vi "Initialize.vi"(7 "Parcel Weight [kg]":dbl, 8 "error in (no error)":errorcluster, 9 "Recipient Data":T1, 10 "Sender Data":T1, 11 "Courier in":refnum<class "Courier.lvclass">) -> (0 "error out":errorcluster, 3 "Courier out":refnum<class "Courier.lvclass">)   [LabVIEW 2019, in "Courier.lvclass"]
uses:
  Courier.lvclass
  C:/Users/Extensa/Desktop/Fabryka/Fabryka Rozwiazanie/Delivery/Delivery/Delivery.lvclass
  Controls/#cluster_PersonalData.ctl
  Delivery/Delivery.lvclass/Delivery.ctl
  Delivery/Delivery.lvclass
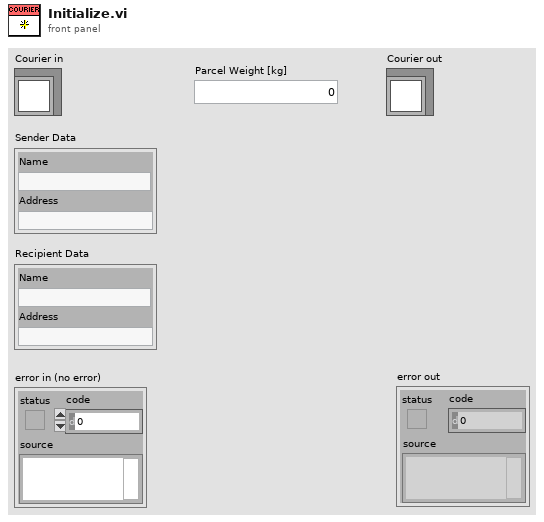
[diagram p1: front panel]
types:
  T1 = typedef "#cluster_PersonalData.ctl" = cluster{"Name":string, "Address":string}
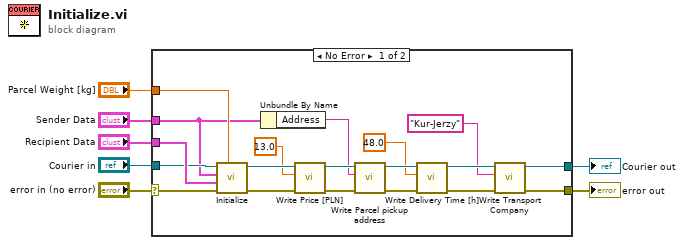
[diagram p0: block diagram]
diagram:
  n1 = case shown="No Error" "error in (no error)" {
    selector: "error in (no error)" -> [w25 w27]
    tunnel: [w8 w27] -> w7
    tunnel: [w9 w28] -> w6
    tunnel: "Parcel Weight [kg]" -> [w26 _]
    tunnel: "Recipient Data" -> [w24 _]
    tunnel: "Sender Data" -> [w17 _]
    tunnel: "Courier in" -> [w23 w28]
    frame No Error {
      n2 = call-parent "Initialize.vi"("Parcel Weight [kg]"=w26, "error in (no error)"=w25, "Recipient Data"=w24, "Sender Data"=w17, "Delivery in"=w23) -> ("error out"=w21:errorcluster, "Delivery out"=w22:refnum<class "Courier.lvclass">)  [unwired: 5 in]
      n3 = Unbundle By Name(w17) -> ("Address"=w16:string)
      n4 = call "Write Price [PLN].vi"("error in (no error)"=w21, "Price [PLN]"=13.0, "Delivery in"=w22) -> ("error out"=w18:errorcluster, "Delivery out"=w19:refnum<class "Courier.lvclass">)  [unwired: 7 in]
      n5 = call "Write Parcel pickup address.vi"("error in (no error)"=w18, "Parcel pickup address"=w16, "Delivery in"=w19) -> ("error out"=w14:errorcluster, "Delivery out"=w15:refnum<class "Courier.lvclass">)  [unwired: 7 in]
      n6 = call "Write Delivery Time [h].vi"("error in (no error)"=w14, "Delivery Time [h]"=48.0, "Delivery in"=w15) -> ("error out"=w12:errorcluster, "Delivery out"=w11:refnum<class "Courier.lvclass">)  [unwired: 7 in]
      n7 = call "Write Transport Company.vi"("error in (no error)"=w12, "Transport Company"="Kur-Jerzy", "Delivery in"=w11) -> ("error out"=w8:errorcluster, "Delivery out"=w9:refnum<class "Courier.lvclass">)  [unwired: 7 in]
    }
    frame Error {
    }
  }
  "error out" <- w7
  "Courier out" <- w6
